vi "PDHSwitchCommandState.vi"(0 "Device Reference (in)":u8=1, 5 "Output Mode":T1(ring), 9 "State [True, False]":bool) -> ()   [LabVIEW 2020]
doc: "Wrapper for commanding the state of a REV PDH switchable port. Supports the standard actuator testing interface and only sending commands on change."
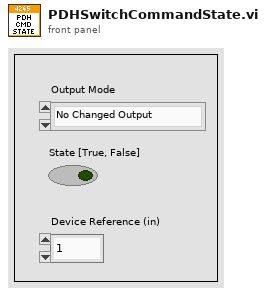
[diagram p1: front panel]
types:
  T1 = enum16{"No Changed Output", "New Normal Output", "New Testing Output"}
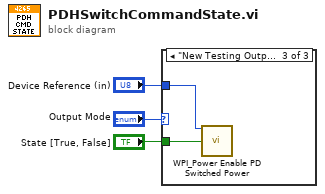
[diagram p0: block diagram]
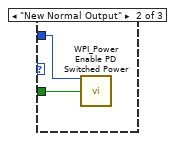
[diagram p3: hidden frame]
diagram:
  n1 = case shown="\"New Testing Output\"" "Output Mode" {
    tunnel: "State [True, False]" -> [_ w5 w7]
    tunnel: "Device Reference (in)" -> [_ w4 w6]
    frame "No Changed Output", Default {
    }
    frame "New Normal Output" {
      n2 = call <vilib>:"WPI_Power Enable PD Switched Power.vi"("Power Distribution (def)"=w4, "Switch Channel Value"=w5) -> ()  [unwired: 12 in, 2 out]
    }
    frame "New Testing Output" {
      n3 = call <vilib>:"WPI_Power Enable PD Switched Power.vi"("Power Distribution (def)"=w6, "Switch Channel Value"=w7) -> ()  [unwired: 12 in, 2 out]
    }
  }
